vi "HeaderAction.vi"(0 "Device en entrée":refnum<class "BaseDevice.lvclass"> caption="DNL_LabVIEW Object in", 11 "error in (no error)":errorcluster caption="entrée d'erreur (pas d'erreur)") -> (4 "Device en sortie":refnum<class "BaseDevice.lvclass"> caption="DNL_LabVIEW Object out", 6 "DataNames":string[](array[string]), 8 "Instr Name":string, 10 "HeaderString":string, 13 "ArrDatNames":string[](array[string]), 14 "DisplayNames":string[](array[string]), 15 "error out":errorcluster caption="sortie d'erreur")   [LabVIEW 2019, in "BaseDevice.lvclass"]
uses:
  BaseDevice.lvclass
  BaseDevice.lvclass/BaseDevice.ctl
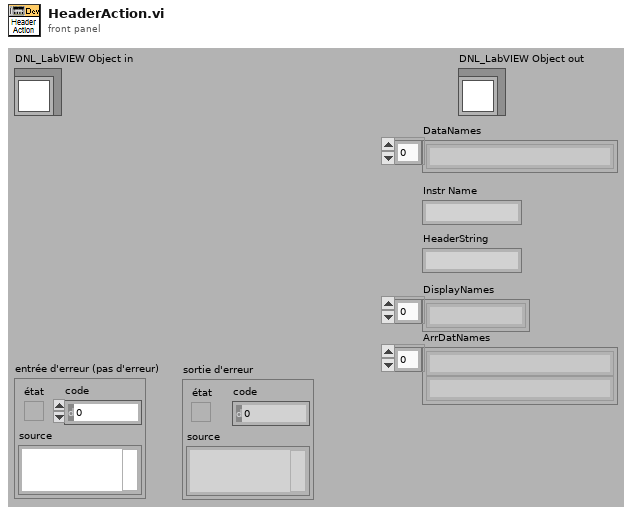
[diagram p1: front panel]
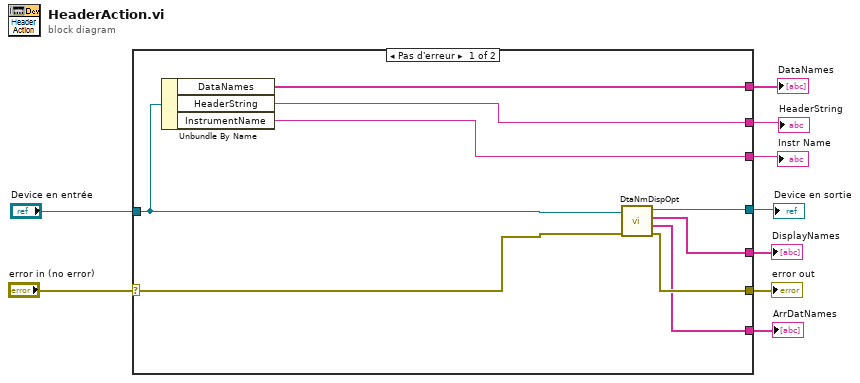
[diagram p0: block diagram]
diagram:
  n1 = case shown="Pas d'erreur" "error in (no error)" {
    selector: "error in (no error)" -> [w11 w20]
    tunnel: [w13 w20] -> w8
    tunnel: [w17 _] -> w7
    tunnel: [w18 _] -> w6
    tunnel: [w16 _] -> w5
    tunnel: [w15 _] -> w4
    tunnel: "Device en entrée" -> [w12 w19]
    tunnel: [w14 w19] -> w2
    tunnel: [w10 _] -> w1
    frame No Error {
      n2 = Unbundle By Name(w12) -> ("DataNames"=w17:string[], "HeaderString"=w18:string, "InstrumentName"=w16:string)
      n3 = call "DtaNmDispOpt.vi"("error in (no error)"=w11, "BaseDevice en entrée"=w12) -> ("error out"=w13:errorcluster, "ArrDisplayNames"=w10:string[], "DisplayNames"=w15:string[], "BaseDevice en sortie"=w14:refnum<class "BaseDevice.lvclass">)  [unwired: 6 in]
    }
    frame Error {
    }
  }
  "error out" <- w8
  "Device en sortie" <- w2
  "DataNames" <- w7
  "HeaderString" <- w6
  "Instr Name" <- w5
  "DisplayNames" <- w4
  "ArrDatNames" <- w1
